vi "BRig_RT__Case_Exp__recordAnalogInput__PortA__dataQ.vi"(0 "input_dataAnalog":u16[][](array[numeric]), 1 "input_index":i32, 2 "input_iOccurence":u16, 3 "resetOccurrence":bool, 4 "input_dataCurrent":u16[](array[numeric]), 5 "input_stateList_NoInterrupt":u16[](array[numeric]), 6 "input_iState_start":T1, 7 "input_dataQ_hdl":refnum<queue>, 8 "input_iState_end":T1, 9 "input_dataQ_error":errorcluster, 10 "input_AI1":u16, 12 "input_AI0":u16) -> (11 "output_dataQ_error":errorcluster, 13 "output_dataQ_hdl":refnum<queue>, 14 "output_dataAnalog":u16[][](array[numeric]), 15 "output_index":i32, 16 "output_iOccurrence":u16)   [LabVIEW 2014]
uses:
  myRIO_BRig_RT__Case_Exp_stateList.ctl
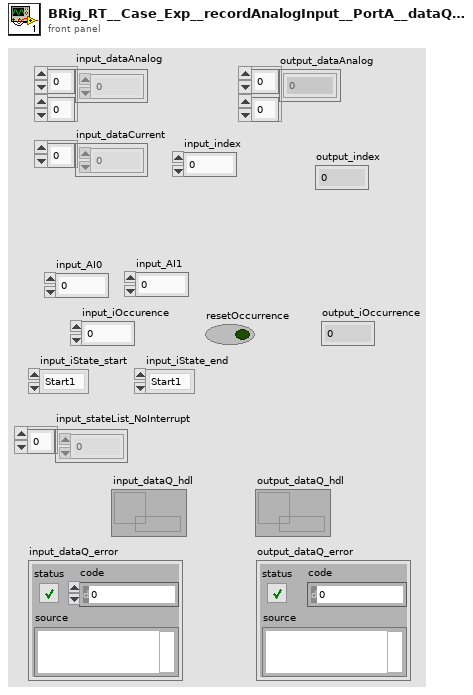
[diagram p1: front panel]
types:
  T1 = typedef "myRIO_BRig_RT__Case_Exp_stateList.ctl" = enum16{"Start1", "Start2", "Start3", "saveSettings1", "saveSettings2", "saveSettings3", "saveSettings4", "saveSettings_LC_ENL_l1", "saveSettings_LC_ENL_l2", "saveSettings_LC_Cue_l1", "saveSettings_LC_Cue_l2", "saveSettings6_LC_l1_Other", "SaveSettings6_LC_l2_Other", "setSettings_Audio", "setSettings_Laser", "initBlock_pre", "initBlock", "initBlock2", "initBlock_post", "initTrial_pre", "initTrial", "initTrial2", "initTrial3", "initTrial4", "initTrial_LC_ENL1", "initTrial_LC_Cue1", "initTrial_LC_Cue1_2", "initTrial_LC_Sel", "initTrial_post", "ENL1_pre", "ENL1", "ENL1_post", "ENL1Penalty_pre", "ENL1Penalty", "ENL2_pre", "ENL2", "ENL2Penalty_pre", "ENL2Penalty", "Cue1_pre", "Cue1", "Cue1_post", "Cue1Penalty_pre", "Cue1Penalty", "Cue2_pre", "Cue2", "Cue2Penalty_pre", "Cue2Penalty", "Selection_pre", "Selection", "Select_post", "SelectReward_pre", "SelectReward", "SelectRewardPost_pre", "SelectRewardPost", "SelectWrong_pre", "SelectWrong", "SelectWrong_post", "SelectTimeout_pre", "SelectTimeout", "SelectTimeout_post", "endTrial_pre", "endTrial1", "endTrial2", "endTrial3", "endTrial_post", "endBlock_pre", "endBlock", "endBlock_post", "endExp", "commConnect", "commUpload_pre", "commUpload_dataBlock", "commUpload_dataCurrent", "commUpload_dataExp", "commUpload_dataLC", "commUpload_dataTrial", "commUpload_post", "saveData_pre", "saveData_dataBlock", "saveData_dataCurrent", "saveData_dataExp", "saveData_dataLC", "saveData_dataTrial", "saveData_post", "empty_endBlock1", "empty_endBlock2", "empty_endTrial1", "empty_endTrial2", "empty_endTrial3", "empty_endTrial4", "empty_endTrial5", "dummyState", "dummyState_endBlock", "FreeReward_pre", "FreeReward", "FreeRewardPost_pre", "FreeRewardPost"}
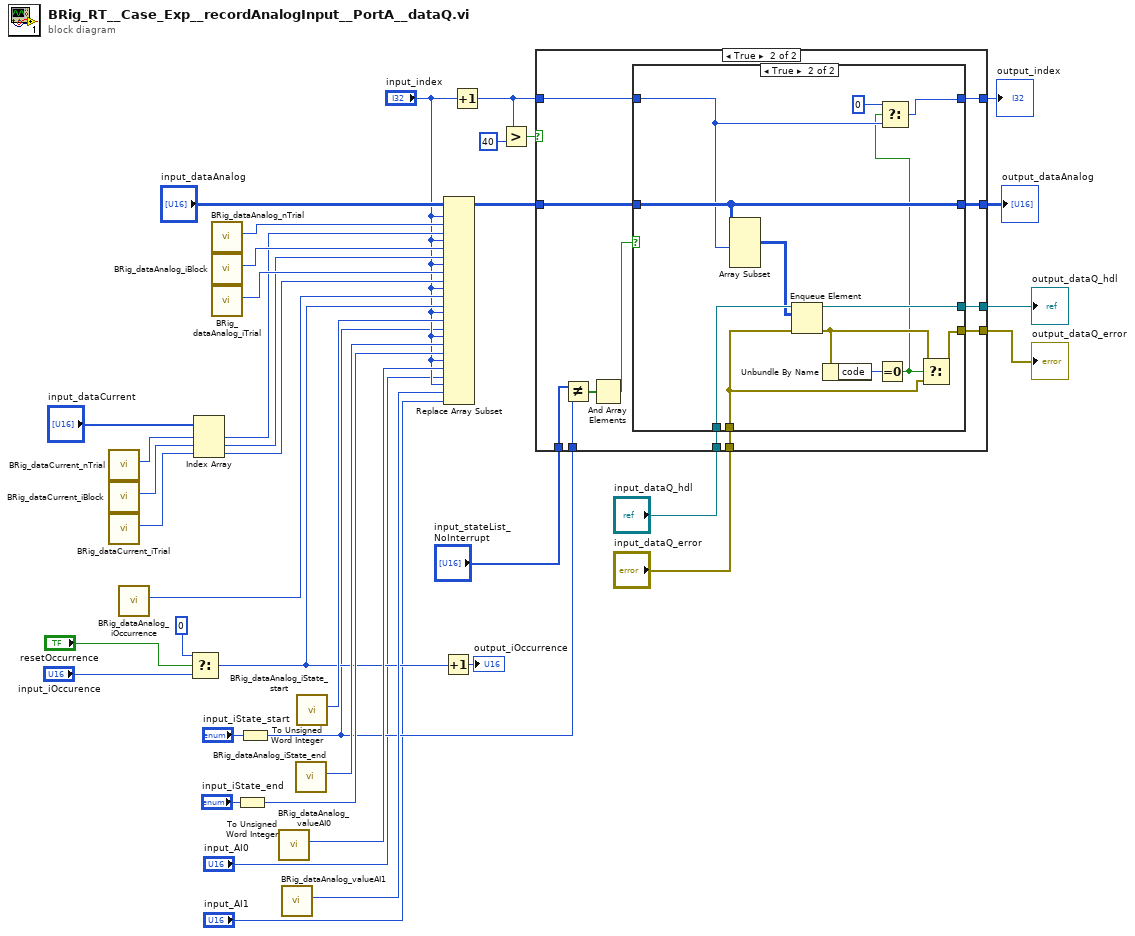
[diagram p0: block diagram]
diagram:
  n1 = call "BRig_dataCurrent_nTrial.vi"() -> ("output_nTrial"=w37:i32)  [unwired: 11 in]
  n2 = call "BRig_dataCurrent_iBlock.vi"() -> ("output_iBlock"=w36:i32)  [unwired: 11 in]
  n3 = call "BRig_dataCurrent_iTrial.vi"() -> ("output_iTrial"=w35:i32)  [unwired: 11 in]
  n4 = call "BRig_dataAnalog_iOccurrence.vi"() -> ("output_iOccurrence"=w28:i32)  [unwired: 11 in]
  n5 = Select(t=u16 0, s="resetOccurrence", f="input_iOccurence") -> (s? t:f=w21:u16)
  n6 = Index Array(array="input_dataCurrent", index #1=w37, index #2=w36, index #3=w35) -> (element #1=w17:u16, element #2=w18:u16, element #3=w16:u16)
  n7 = call "BRig_dataAnalog_nTrial.vi"() -> ("output_nTrial"=w34:i32)  [unwired: 11 in]
  n8 = call "BRig_dataAnalog_iBlock.vi"() -> ("output_iBlock"=w33:i32)  [unwired: 11 in]
  n9 = call "BRig_dataAnalog_iTrial.vi"() -> ("output_iTrial"=w32:i32)  [unwired: 11 in]
  n10 = To Unsigned Word Integer(number="input_iState_end") -> (unsigned 16bit integer=w27:u16)
  n11 = To Unsigned Word Integer(number="input_iState_start") -> (unsigned 16bit integer=w8:u16)
  n12 = call "BRig_dataAnalog_valueAI0.vi"() -> ("output_valueAI0"=w26:i32)  [unwired: 11 in]
  n13 = call "BRig_dataAnalog_valueAI1.vi"() -> ("output_valueAI1"=w25:i32)  [unwired: 11 in]
  n14 = call "BRig_dataAnalog_iState_end.vi"() -> ("output_iState_end"=w29:i32)  [unwired: 11 in]
  n15 = call "BRig_dataAnalog_iState_start.vi"() -> ("output_iState_start"=w30:i32)  [unwired: 11 in]
  n16 = Increment(x=w21) -> (x+1=→"output_iOccurrence":u16)
  n17 = Replace Array Subset(array="input_dataAnalog", new element #1=w17, index (row) #1="input_index", index (col) #1=w34, new element #2=w18, index (row) #2="input_index", index (col) #2=w33, new element #3=w16, index (row) #3="input_index", index (col) #3=w32, new element #4=w21, index (row) #4="input_index", index (col) #4=w28, new element #5=w8, index (row) #5="input_index", index (col) #5=w30, new element #6=w27, index (row) #6="input_index", index (col) #6=w29, new element #7="input_AI0", index (row) #7="input_index", index (col) #7=w26, new element #8="input_AI1", index (row) #8="input_index", index (col) #8=w25) -> (w12:u16[][])
  n18 = Increment(x="input_index") -> (x+1=w11:i32)
  n19 = Greater?(x=w11, y=40) -> (0:w13:bool)
  n20 = case shown="True" w13 {
    tunnel: w12 -> [w43 w54]
    tunnel: [w43 w54] -> w10
    tunnel: w11 -> [w42 w53]
    tunnel: [w42 w52] -> w9
    tunnel: w8 -> [_ w50]
    tunnel: "input_stateList_NoInterrupt" -> [_ w51]
    tunnel: "input_dataQ_hdl" -> [w41 w47]
    tunnel: "input_dataQ_error" -> [w40 w46]
    tunnel: [w41 w45] -> w4
    tunnel: [w40 w44] -> w3
    frame False {
    }
    frame True {
      n21 = Not Equal?(x=w51, y=w50) -> (x != y?=w49:bool[])
      n22 = And Array Elements(Boolean array=w49) -> (logical AND=w48:bool)
      n23 = case shown="True" w48 {
        tunnel: w54 -> [w57 w67]
        tunnel: w53 -> [w58 w70]
        tunnel: [w58 w68] -> w52
        tunnel: [w57 w67] -> _
        tunnel: w47 -> [w55 w66]
        tunnel: w46 -> [w56 w60]
        tunnel: [w55 w64] -> w45
        tunnel: [w56 w61] -> w44
        frame False {
        }
        frame True {
          n24 = Array Subset(array=w67, length (row)=w70) -> (w65:u16[][])  [unwired: 3 in]
          n25 = Enqueue Element(queue=w66, element=w65, error in (no error)=w60) -> (queue out=w64:refnum<queue>, error out=w62:errorcluster)  [unwired: 1 in, 1 out]
          n26 = Unbundle By Name(w62) -> ("code"=w63:i32)
          n27 = Equal To 0?(x=w63) -> (x = 0?=w59:bool)
          n28 = Select(t=0, s=w59, f=w70) -> (s? t:f=w68:i32)
          n29 = Select(t=w62, s=w59, f=w60) -> (s? t:f=w61:errorcluster)
        }
      }
    }
  }
  "output_dataAnalog" <- w10
  "output_index" <- w9
  "output_dataQ_hdl" <- w4
  "output_dataQ_error" <- w3
